vi "InitializeSession.vi"(8 "error in (no error)":errorcluster, 10 "Initialize_Session":variant, 11 "NI-DMM in":refnum<class "NI-DCPower.lvclass">) -> (0 "error out":errorcluster, 3 "NI-DMM out":refnum<class "NI-DCPower.lvclass">)   [LabVIEW 2020, in "NI-DCPower.lvclass"]
uses:
  NI-DCPower.lvclass
  C:/Program Files/National Instruments/LabVIEW 2020/vi.lib/MeasurementLink/MeasurementLink Instrument/ISession Factory/ISession Factory.lvclass
  NI-DCPower.lvclass/NI-DCPower.ctl
  98def37a-749e-46e7-8016-72a2eaa208e4.vi
  <vilib>/MeasurementLink/MeasurementLink Session Management V1/Session Reservation/Initialize Sessions with Retry.vi
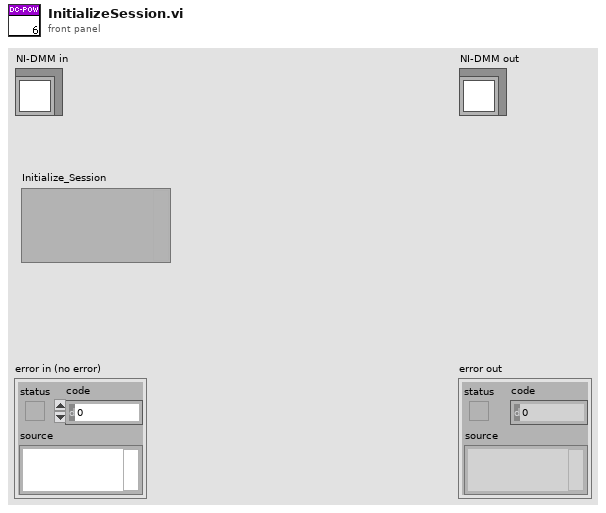
[diagram p1: front panel]
types:
  T1 = typedef "NI-DCPower.lvclass/Initialize_Info.ctl" = cluster{"initialize and close session behavior":T2, "reset":bool, "optional string":string}
  T2 = typedef "MeasurementLink Session Management V1.lvlib/Session Reservation.lvclass/Initialize and Close Session Behavior.ctl" = enum16{"Auto", "Initialize and Close", "Attach and Detach", "Initialize and Detach", "Attach and Close"}
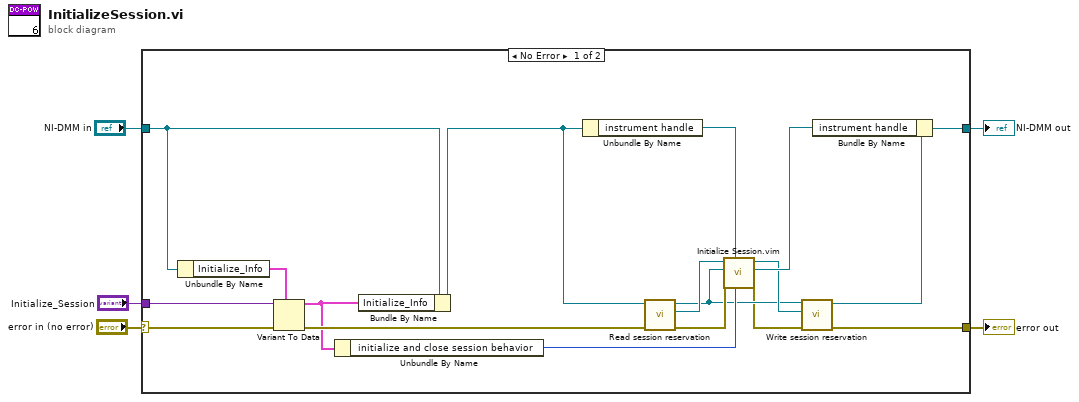
[diagram p0: block diagram]
diagram:
  n1 = case shown="No Error" "error in (no error)" {
    selector: "error in (no error)" -> [w21 w25]
    tunnel: "Initialize_Session" -> [w20 _]
    tunnel: "NI-DMM in" -> [w19 w24]
    tunnel: [w8 w25] -> w2
    tunnel: [w14 w24] -> w1
    frame No Error {
      n2 = Unbundle By Name(w19) -> ("Initialize_Info"=w18:T1)
      n3 = Variant To Data(error in=w21, type=w18, Variant=w20) -> (data=w6:T1, error out=w15:errorcluster)
      n4 = Unbundle By Name(w6) -> ("initialize and close session behavior"=w17:T2)
      n5 = Bundle By Name(cluster=w19, "Initialize_Info"=w6) -> (w7:refnum<class "NI-DCPower.lvclass">)
      n6 = Unbundle By Name(w7) -> ("instrument handle"=w23:refnum<k15>)
      n7 = call-dynamic "Read session reservation.vi"("error in (no error)"=w15, "Abstract_Instrument in"=w7) -> ("error out"=w16:errorcluster, "Session Reservation.lvclass"=w22:refnum<class "Session Reservation.lvclass">, "Abstract_Instrument out"=w11:refnum<class "NI-DCPower.lvclass">)  [unwired: 7 in]
      n8 = call "Initialize Session.vim"("initialize and close session behavior"=w17, "session type"=w23, "error in"=w16, "session factory"=w11, "session reservation in"=w22) -> ("error out"=w9:errorcluster, "session"=w13:refnum<k15>, "session reservation out"=w12:refnum<class "Session Reservation.lvclass">)  [unwired: 3 in, 1 out]
      n9 = call-dynamic "Write session reservation.vi"("error in (no error)"=w9, "Session Reservation.lvclass"=w12, "Abstract_Instrument in"=w11) -> ("error out"=w8:errorcluster, "Abstract_Instrument out"=w10:refnum<class "NI-DCPower.lvclass">)  [unwired: 7 in]
      n10 = Bundle By Name(cluster=w10, "instrument handle"=w13) -> (w14:refnum<class "NI-DCPower.lvclass">)
    }
    frame Error {
    }
  }
  "error out" <- w2
  "NI-DMM out" <- w1
